vi "shutterGetList.vi"() -> (0 "list of shutters":i32[](array[numeric]))   [LabVIEW 2017]
uses:
  globalDevices.vi
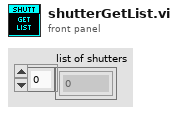
[diagram p1: front panel]
types:
  T1 = cluster{"serialPort":refnum<visa-resource-name>, "error":errorcluster, "power (mW)":dbl, "wavelength (nm)":dbl, "type":string, "shutter":i32}[]
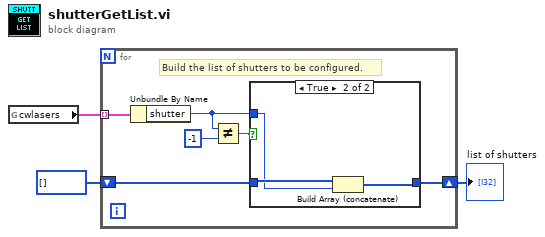
[diagram p0: block diagram]
diagram:
  n1 = global read "globalDevices.vi" "cwlasers"() -> (w3:T1)
  n2 = for {
    tunnel: w3 -> [w9] mode=indexing
    shift-right: [w4] -> w1
    shift-left: i32[] [] -> [w5]
    # "Build the list of shutters to be configured."
    n3 = Unbundle By Name(w9) -> ("shutter"=w6:i32)
    n4 = Not Equal?(x=w6, y=-1) -> (x != y?=w7:bool)
    n5 = case shown="True" w7 {
      tunnel: w6 -> [_ w12]
      tunnel: w5 -> [w10 w13]
      tunnel: [w10 w11] -> w4
      frame False {
      }
      frame True {
        n6 = Build Array (concatenate)(w13, w12) -> (w11:i32[])
      }
    }
  }
  "list of shutters" <- w1
